vi "总磷总氮测量数据储存.vi"() -> ()   [LabVIEW 2022 SP3, in "斯坦道CODcr.lvlib"]
uses:
  <vilib>/ptbypt/NI_PtbyPt.lvlib
panel:
  in  "x":bool
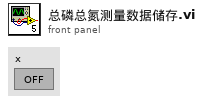
[diagram p1: front panel]
types:
  T1 = cluster{"跨度值":dbl, "零点标准液浓度":dbl, "跨度标准液浓度":dbl, "标准液标准浓度":dbl}
  T2 = cluster{"系统时间":timestamp, "工作状态":u16, "测量模式":enum16{"待机", "连续模式", "周期模式", "定点模式", "受控模式", "手动模式"}, "告警代码":u16, "故障代码":u16, "日志代码":u16, "软件版本":u16, "F0":sgl, "F1":sgl, "F2":sgl, "F3":sgl, "T":sgl, "H":sgl, "id":u16, "flowid":u16, "量程":u16, "总磷控温温度1":sgl, "营养盐控温温度2":sgl, "ADC":sgl, "结果值":sgl, "运行时间":u16, "步骤详情":string, "步骤流程":string}
  T3 = cluster{"运行模式":enum16{"维护模式", "常规模式", "应急模式", "质控模式", "性能测试"}, "质控频次":enum16{"关闭", "每天", "星期一", "星期二", "星期三", "星期四", "星期五", "星期六", "星期日"}, "空白核查时间":u16, "跨度核查时间":u16, "测量间隔":u16}
  T4 = cluster{"测量精度":u16, "消解温度":u16, "消解时长":u16, "量程下限":sgl, "量程上限":sgl, "曲线斜率K":sgl, "曲线斜率B":sgl, "标定日期":timestamp, "标液1浓度":sgl, "标液1测量过程值":sgl, "标液2浓度":sgl, "标液2测量过程值":sgl, "标液3浓度":sgl, "标液3测量过程值":sgl, "标液4浓度":sgl, "标液4测量过程值":sgl, "标液5浓度":sgl, "标液5测量过程值":sgl, "线性相关系数":sgl, "试剂余量":u32, "测量滴定值或吸光度":sgl, "空白校准时间":timestamp, "标样校准时间":timestamp, "检出限值":sgl, "校准系数":sgl, "设备系列号":string}[]
  T5 = cluster{"因子编码":u32, "单位":u16, "标样参考值":sgl, "水样数据时间":timestamp, "水样实测值":sgl, "水样数据标识":string, "标样数据时间":timestamp, "标样实测值":sgl, "标样数据标识":string, "空白数据时间":timestamp, "空白实测值":sgl, "空白数据标识":string, "零点核查数据时间":timestamp, "零点核查实测值":sgl, "零点核查数据标识":string, "跨度核查数据时间":timestamp, "跨度核查实测值":sgl, "跨度核查数据标识":string, "加标回收数据时间":timestamp, "加标回收实测值":sgl, "加标回收数据标识":string, "平行样数据时间":timestamp, "平行样实测值":sgl, "平行样数据标识":string, "F0":sgl, "F1":sgl, "F2":sgl, "F3":sgl, "F4":sgl, "F5":sgl, "F6":sgl, "F7":sgl, "温度":sgl, "湿度":sgl, "X值":sgl, "fidrange":u16, "X1值":sgl}[]
  T6 = cluster{"总磷跨度值":dbl, "总磷零点标准液浓度":dbl, "总磷跨度标准液浓度":dbl, "总磷标准液标准浓度":dbl, "总氮跨度值":dbl, "总氮零点标准液浓度":dbl, "总氮跨度标准液浓度":dbl, "总氮标准液标准浓度":dbl, "COD跨度值":dbl, "COD零点标准液浓度":dbl, "COD跨度标准液浓度":dbl, "COD标准液标准浓度":dbl, "氨氮跨度值":dbl, "氨氮零点标准液浓度":dbl, "氨氮跨度标准液浓度":dbl, "氨氮标准液标准浓度":dbl, "磷酸盐跨度值":dbl, "磷酸盐零点标准液浓度":dbl, "磷酸盐跨度标准液浓度":dbl, "磷酸盐标准液标准浓度":dbl, "硝氮跨度值":dbl, "硝氮零点标准液浓度":dbl, "硝氮跨度标准液浓度":dbl, "硝氮标准液标准浓度":dbl, "亚硝氮跨度值":dbl, "亚硝氮零点标准液浓度":dbl, "亚硝氮跨度标准液浓度":dbl, "亚硝氮标准液标准浓度":dbl, "硫化物跨度值":dbl, "硫化物零点标准液浓度":dbl, "硫化物跨度标准液浓度":dbl, "硫化物标准液标准浓度":dbl, "硅酸盐跨度值":dbl, "硅酸盐零点标准液浓度":dbl, "硅酸盐跨度标准液浓度":dbl, "硅酸盐标准液标准浓度":dbl, "总磷零点标准液偏差":dbl, "总磷跨度标准液偏差":dbl, "总磷标准液标准偏差":dbl, "总氮零点标准液偏差":dbl, "总氮跨度标准液偏差":dbl, "总氮标准液标准偏差":dbl, "COD零点标准液偏差":dbl, "COD跨度标准液偏差":dbl, "COD标准液标准偏差":dbl, "氨氮零点标准液偏差":dbl, "氨氮跨度标准液偏差":dbl, "氨氮标准液标准偏差":dbl, "磷酸盐零点标准液偏差":dbl, "磷酸盐跨度标准液偏差":dbl, "磷酸盐标准液标准偏差":dbl, "硝氮零点标准液偏差":dbl, "硝氮跨度标准液偏差":dbl, "硝氮标准液标准偏差":dbl, "亚硝氮零点标准液偏差":dbl, "亚硝氮跨度标准液偏差":dbl, "亚硝氮标准液标准偏差":dbl, "硫化物零点标准液偏差":dbl, "硫化物跨度标准液偏差":dbl, "硫化物标准液标准偏差":dbl, "硅酸盐零点标准液偏差":dbl, "硅酸盐跨度标准液偏差":dbl, "硅酸盐标准液标准偏差":dbl, "氟化物跨度值":dbl, "氟化物零点标准液浓度":dbl, "氟化物跨度标准液浓度":dbl, "氟化物标准液标准浓度":dbl, "氟化物零点标准液偏差":dbl, "氟化物跨度标准液偏差":dbl, "氟化物标准液标准偏差":dbl, "CODMn跨度值":dbl, "CODMn零点标准液浓度":dbl, "CODMn跨度标准液浓度":dbl, "CODMn标准液标准浓度":dbl, "CODMn零点标准液偏差":dbl, "CODMn跨度标准液偏差":dbl, "CODMn标准液标准偏差":dbl}
  T7 = enum16{"水样测试", "标样核查", "跨度核查", "零点核查", "加标回收", "空白测试", "平行样"}[]
  T8 = cluster{"因子编码":u32, "单位":u16, "标样参考值":sgl, "水样数据时间":timestamp, "水样实测值":sgl, "水样数据标识":string, "标样数据时间":timestamp, "标样实测值":sgl, "标样数据标识":string, "空白数据时间":timestamp, "空白实测值":sgl, "空白数据标识":string, "零点核查数据时间":timestamp, "零点核查实测值":sgl, "零点核查数据标识":string, "跨度核查数据时间":timestamp, "跨度核查实测值":sgl, "跨度核查数据标识":string, "加标回收数据时间":timestamp, "加标回收实测值":sgl, "加标回收数据标识":string, "平行样数据时间":timestamp, "平行样实测值":sgl, "平行样数据标识":string, "F0":sgl, "F1":sgl, "F2":sgl, "F3":sgl, "F4":sgl, "F5":sgl, "F6":sgl, "F7":sgl, "温度":sgl, "湿度":sgl, "X值":sgl, "fidrange":u16, "X1值":sgl}
  T9 = cluster{"时间标识":timestamp, "测量模式":enum16{"维护数据", "水样测试", "标样核查", "零点核查", "跨度核查", "空白测试", "平行样测试", "加标回收", "空白校准", "标样校准", "初始化（清洗）", "快捷测试"}, "数据标记表":string, "监测值":sgl, "单位":u16, "数据标识":string, "因子编码":u32, "标样参考值":sgl, "F0":sgl, "F1":sgl, "F2":sgl, "F3":sgl, "F4":sgl, "F5":sgl, "F6":sgl, "F7":sgl, "X":sgl, "温度":sgl, "湿度":sgl, "量程标识":string, "SN":string, "跨度值":sgl, "X1":sgl}
  T10 = typedef "斯坦道CODcr.lvlib/关键参数.ctl" = cluster{"测量量程":sgl, "测量检出限":sgl, "测量精度":sgl, "测量间隔":sgl, "消解温度":sgl, "消解时长":sgl, "三项式系数":sgl, "二次多项式系数":sgl, "曲线斜率":sgl, "曲线截距":sgl, "线性相关系数":sgl, "空白校准时间":timestamp, "标样校准时间":timestamp, "测量信号值":sgl, "稀释倍数":sgl, "空白标定系数":sgl, "量程系数":sgl}
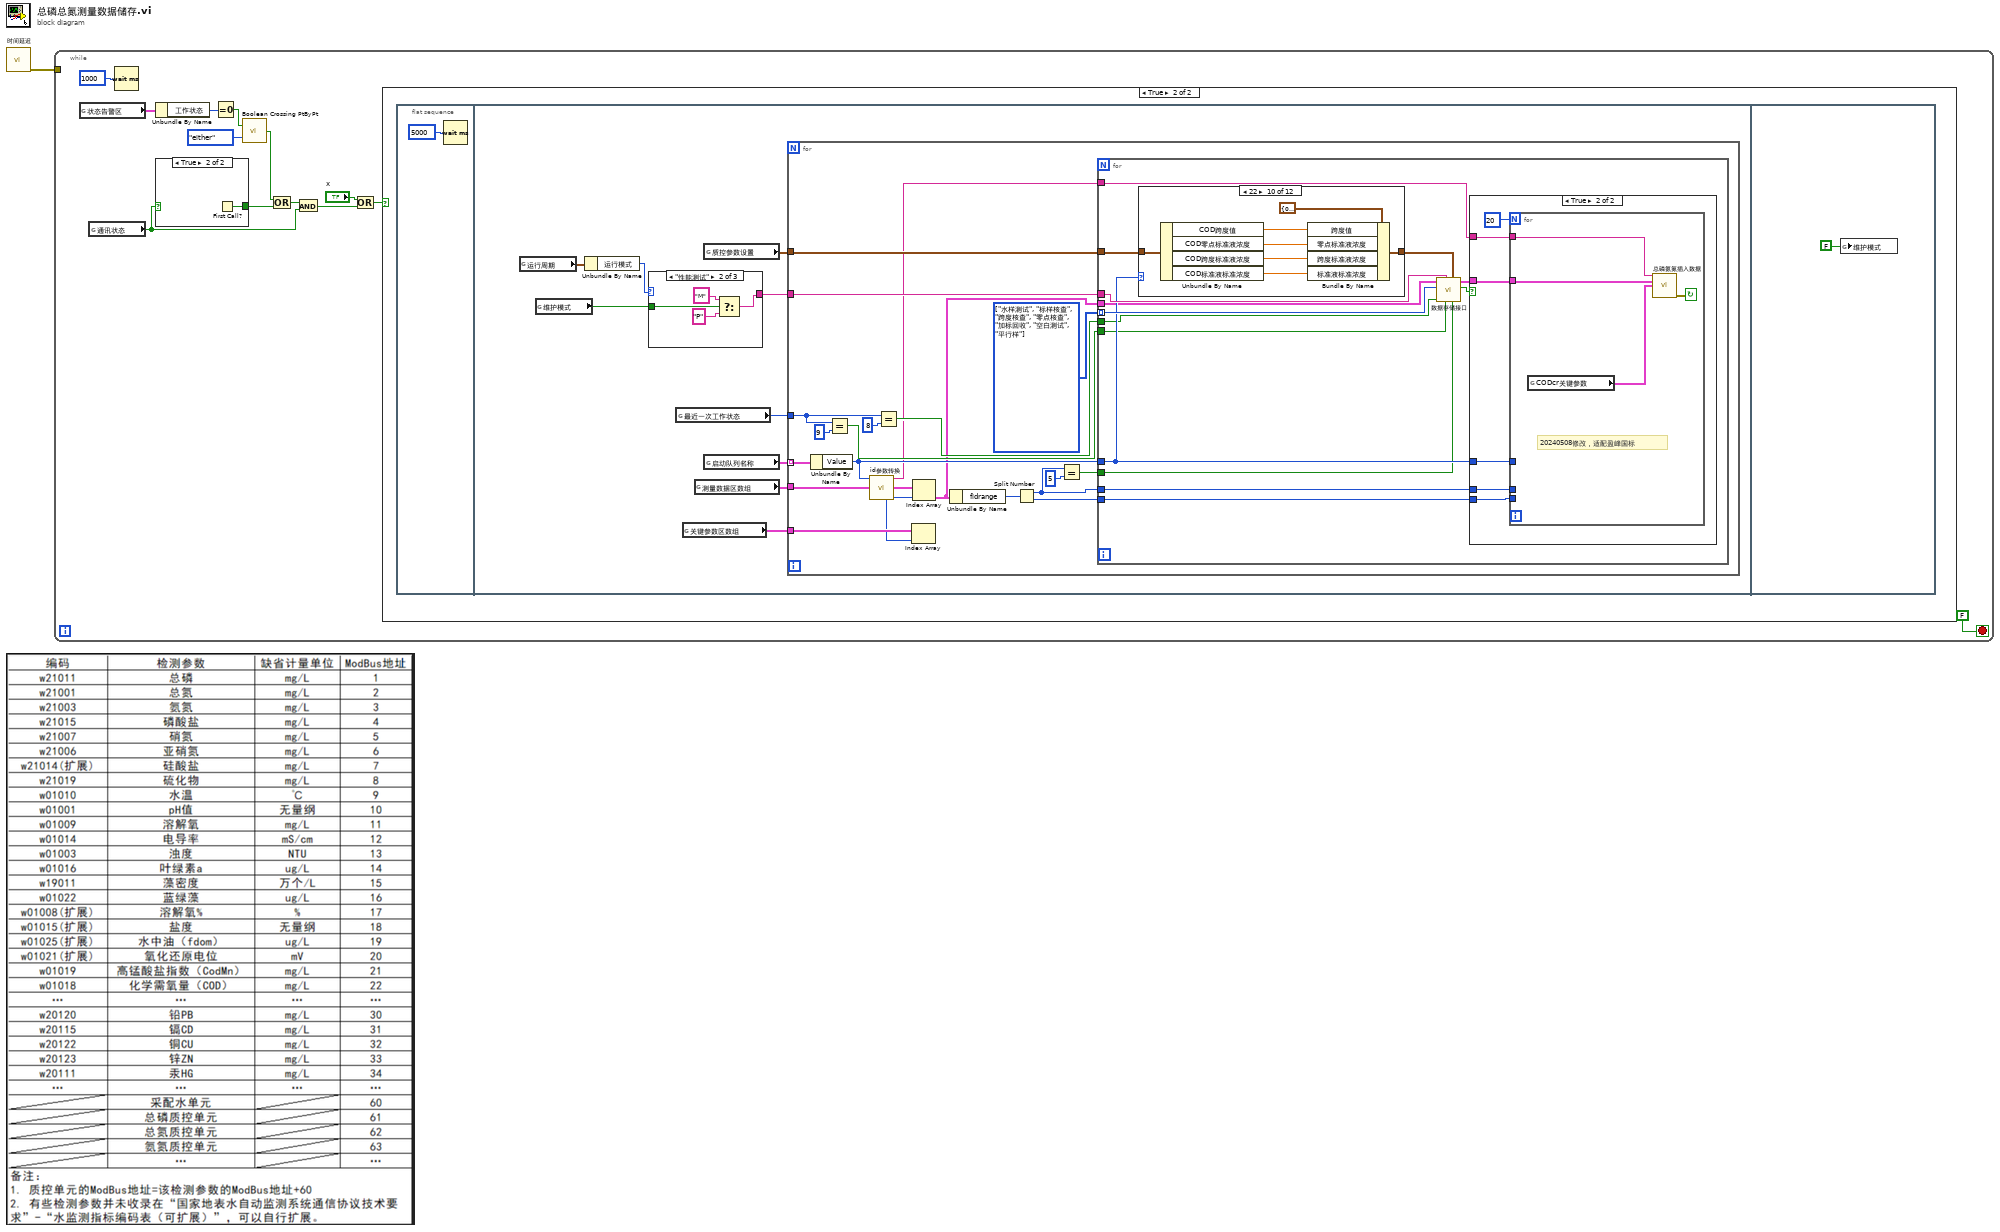
[diagram p0: block diagram]
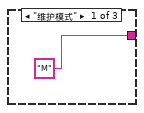
[diagram p4: hidden frame]
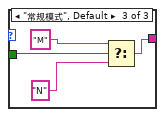
[diagram p5: hidden frame]
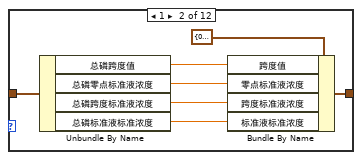
[diagram p8: hidden frame]
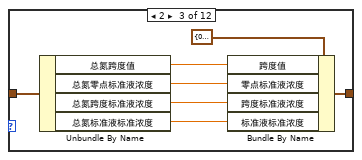
[diagram p9: hidden frame]
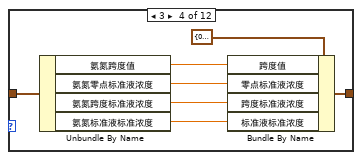
[diagram p10: hidden frame]
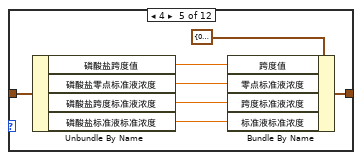
[diagram p11: hidden frame]
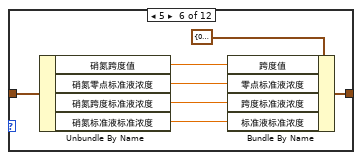
[diagram p12: hidden frame]
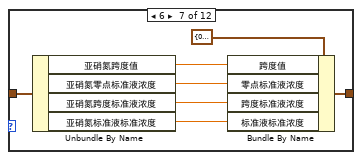
[diagram p13: hidden frame]
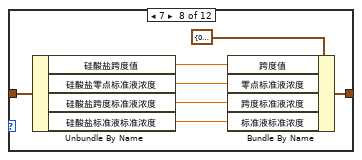
[diagram p14: hidden frame]
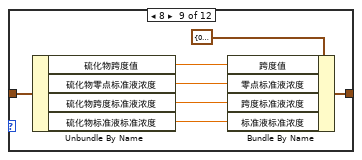
[diagram p15: hidden frame]
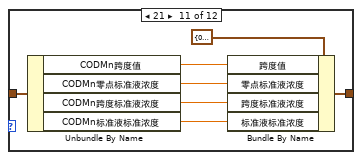
[diagram p16: hidden frame]
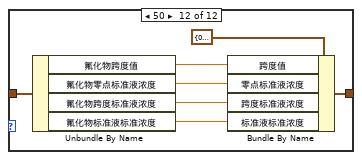
[diagram p17: hidden frame]
diagram:
  n1 = call "时间延迟"() -> ("error out"=w1:errorcluster)  [unwired: 11 in]
  n2 = while {
    tunnel: w1 -> [_]
    stop <- FALSE stop-if-true
    n3 = global read "VAR总磷总氮全局变量.vi" "状态告警区"() -> (w13:T2)
    n4 = global read "VAR总磷总氮全局变量.vi" "通讯状态"() -> (w6:bool)
    n5 = Wait (ms)(milliseconds to wait=u32 1000 ("等待时间（毫秒）")) -> ()  [unwired: 1 out]
    n6 = Unbundle By Name(w13) -> ("工作状态"=w11:u16)
    n7 = case shown="True" w6 {
      tunnel: [_ w15] -> w4
      frame False {
      }
      frame True {
        n8 = First Call?() -> (First Call?: T/F=w15:bool)
      }
    }
    n9 = Equal To 0?(x=w11) -> (x = 0?=w8:bool)
    n10 = call <vilib>:"Boolean Crossing PtByPt.vi"("direction"=enum16{"either", "false-true", "true-false"}."either", "input"=w8) -> ("crossing"=w9:bool)  [unwired: 1 in]
    n11 = Or(x=w9, y=w4) -> (x .or. y?=w5:bool)
    n12 = And(x=w5, y=w6) -> (x .and. y?=w7:bool)
    n13 = Or(x="x", y=w7) -> (x .or. y?=w3:bool)
    n14 = case shown="True" w3 {
      frame False {
      }
      frame True {
        n15 = flat-sequence {
          frame #0 {
            n16 = Wait (ms)(milliseconds to wait=u32 5000 ("等待时间（毫秒）")) -> ()  [unwired: 1 out]
          }
          frame #1 {
            n17 = global read "总磷总氮断电保存全局变量.vi" "运行周期"() -> (w22:T3)
            n18 = global read "VAR总磷总氮全局变量.vi" "维护模式"() -> (w19:bool)
            n19 = Unbundle By Name(w22) -> ("运行模式"=w20:enum16{"维护模式", "常规模式", "应急模式", "质控模式", "性能测试"})
            n20 = case shown="\"性能测试\"" w20 {
              tunnel: ["M" w27 w32] -> w21
              tunnel: w19 -> [_ w28 w34]
              frame "维护模式" {
              }
              frame "性能测试" {
                n21 = Select(t="M", s=w28, f="P") -> (s? t:f=w27:string)
              }
              frame "常规模式", Default {
                n22 = Select(t="M", s=w34, f="N") -> (s? t:f=w32:string)
              }
            }
            n23 = global read "VAR总磷总氮全局变量.vi" "最近一次工作状态"() -> (w24:u16)
            n24 = global read "VAR总磷总氮全局变量.vi" "关键参数区数组"() -> (w17:T4)
            n25 = global read "VAR总磷总氮全局变量.vi" "测量数据区数组"() -> (w18:T5)
            n26 = global read "总磷总氮断电保存全局变量.vi" "质控参数设置"() -> (w23:T6)
            n27 = global read "model config var.vi" "启动队列名称"() -> (w25:cluster{"String":string, "Value":u16}[])
            n28 = for {
              tunnel: w25 -> [w51] mode=indexing
              tunnel: w24 -> [w47]
              tunnel: w23 -> [w53]
              tunnel: w21 -> [w52]
              tunnel: w18 -> [w37]
              tunnel: w17 -> [w36]
              w54 = T7 [enum."水样测试", enum."标样核查", enum."跨度核查", enum."零点核查", enum."加标回收", enum."空白测试", enum."平行样"] items=["水样测试", "标样核查", "跨度核查", "零点核查", "加标回收", "空白测试", "平行样"]
              n29 = Unbundle By Name(w51) -> ("Value"=w45:u16)
              n30 = Equal?(x=w47, y=u16 9) -> (x = y?=w46:bool)
              n31 = call "id参数转换.vi"("id"=w45) -> ("table输出"=w44:string, "数组资源索引"=w35:i32)  [unwired: 9 in]
              n32 = Equal?(x=w47, y=u16 8) -> (x = y?=w49:bool)
              n33 = Index Array(array=w36, index=w35) -> ()  [unwired: 1 out]
              n34 = Index Array(array=w37, index=w35) -> (element=w41:T8)
              n35 = Unbundle By Name(w41) -> ("fidrange"=w43:u16)
              n36 = Split Number(x=w43) -> (hi(x)=w38:u8, lo(x)=w39:u8)
              n37 = Equal?(x=w38, y=u16 5) -> (x = y?=w40:bool)
              n38 = for {
                tunnel: w54 -> [w66] mode=indexing
                tunnel: w53 -> [w65]
                tunnel: w52 -> [w64]
                tunnel: w45 -> [w63]
                tunnel: w49 -> [w62]
                tunnel: w46 -> [w61]
                tunnel: w41 -> [w56]
                tunnel: w44 -> [w60]
                tunnel: w40 -> [w59]
                tunnel: w39 -> [w58]
                tunnel: w38 -> [w57]
                n39 = case shown="22" w63 {
                  tunnel: w65 -> [_ w85 w92 w99 w106 w113 w120 w127 w134 w141 w148 w155]
                  tunnel: [_ w83 w90 w97 w104 w111 w118 w125 w132 w139 w146 w153] -> w67
                  frame 0, Default {
                  }
                  frame 1 {
                    n40 = Unbundle By Name(w85) -> ("总磷跨度值"=w82:dbl, "总磷零点标准液浓度"=w81:dbl, "总磷跨度标准液浓度"=w80:dbl, "总磷标准液标准浓度"=w79:dbl)
                    n41 = Bundle By Name(cluster=T1 {"跨度值"=0.0, "零点标准液浓度"=0.0, "跨度标准液浓度"=0.0, "标准液标准浓度"=0.0} ("质控参数设置"), "跨度值"=w82, "零点标准液浓度"=w81, "跨度标准液浓度"=w80, "标准液标准浓度"=w79) -> (w83:T1)
                  }
                  frame 2 {
                    n42 = Unbundle By Name(w92) -> ("总氮跨度值"=w89:dbl, "总氮零点标准液浓度"=w88:dbl, "总氮跨度标准液浓度"=w87:dbl, "总氮标准液标准浓度"=w86:dbl)
                    n43 = Bundle By Name(cluster=T1 {"跨度值"=0.0, "零点标准液浓度"=0.0, "跨度标准液浓度"=0.0, "标准液标准浓度"=0.0} ("质控参数设置"), "跨度值"=w89, "零点标准液浓度"=w88, "跨度标准液浓度"=w87, "标准液标准浓度"=w86) -> (w90:T1)
                  }
                  frame 3 {
                    n44 = Unbundle By Name(w99) -> ("氨氮跨度值"=w96:dbl, "氨氮零点标准液浓度"=w95:dbl, "氨氮跨度标准液浓度"=w94:dbl, "氨氮标准液标准浓度"=w93:dbl)
                    n45 = Bundle By Name(cluster=T1 {"跨度值"=0.0, "零点标准液浓度"=0.0, "跨度标准液浓度"=0.0, "标准液标准浓度"=0.0} ("质控参数设置"), "跨度值"=w96, "零点标准液浓度"=w95, "跨度标准液浓度"=w94, "标准液标准浓度"=w93) -> (w97:T1)
                  }
                  frame 4 {
                    n46 = Unbundle By Name(w106) -> ("磷酸盐跨度值"=w103:dbl, "磷酸盐零点标准液浓度"=w102:dbl, "磷酸盐跨度标准液浓度"=w101:dbl, "磷酸盐标准液标准浓度"=w100:dbl)
                    n47 = Bundle By Name(cluster=T1 {"跨度值"=0.0, "零点标准液浓度"=0.0, "跨度标准液浓度"=0.0, "标准液标准浓度"=0.0} ("质控参数设置"), "跨度值"=w103, "零点标准液浓度"=w102, "跨度标准液浓度"=w101, "标准液标准浓度"=w100) -> (w104:T1)
                  }
                  frame 5 {
                    n48 = Unbundle By Name(w113) -> ("硝氮跨度值"=w110:dbl, "硝氮零点标准液浓度"=w109:dbl, "硝氮跨度标准液浓度"=w108:dbl, "硝氮标准液标准浓度"=w107:dbl)
                    n49 = Bundle By Name(cluster=T1 {"跨度值"=0.0, "零点标准液浓度"=0.0, "跨度标准液浓度"=0.0, "标准液标准浓度"=0.0} ("质控参数设置"), "跨度值"=w110, "零点标准液浓度"=w109, "跨度标准液浓度"=w108, "标准液标准浓度"=w107) -> (w111:T1)
                  }
                  frame 6 {
                    n50 = Unbundle By Name(w120) -> ("亚硝氮跨度值"=w117:dbl, "亚硝氮零点标准液浓度"=w116:dbl, "亚硝氮跨度标准液浓度"=w115:dbl, "亚硝氮标准液标准浓度"=w114:dbl)
                    n51 = Bundle By Name(cluster=T1 {"跨度值"=0.0, "零点标准液浓度"=0.0, "跨度标准液浓度"=0.0, "标准液标准浓度"=0.0} ("质控参数设置"), "跨度值"=w117, "零点标准液浓度"=w116, "跨度标准液浓度"=w115, "标准液标准浓度"=w114) -> (w118:T1)
                  }
                  frame 7 {
                    n52 = Unbundle By Name(w127) -> ("硅酸盐跨度值"=w124:dbl, "硅酸盐零点标准液浓度"=w123:dbl, "硅酸盐跨度标准液浓度"=w122:dbl, "硅酸盐标准液标准浓度"=w121:dbl)
                    n53 = Bundle By Name(cluster=T1 {"跨度值"=0.0, "零点标准液浓度"=0.0, "跨度标准液浓度"=0.0, "标准液标准浓度"=0.0} ("质控参数设置"), "跨度值"=w124, "零点标准液浓度"=w123, "跨度标准液浓度"=w122, "标准液标准浓度"=w121) -> (w125:T1)
                  }
                  frame 8 {
                    n54 = Unbundle By Name(w134) -> ("硫化物跨度值"=w131:dbl, "硫化物零点标准液浓度"=w130:dbl, "硫化物跨度标准液浓度"=w129:dbl, "硫化物标准液标准浓度"=w128:dbl)
                    n55 = Bundle By Name(cluster=T1 {"跨度值"=0.0, "零点标准液浓度"=0.0, "跨度标准液浓度"=0.0, "标准液标准浓度"=0.0} ("质控参数设置"), "跨度值"=w131, "零点标准液浓度"=w130, "跨度标准液浓度"=w129, "标准液标准浓度"=w128) -> (w132:T1)
                  }
                  frame 22 {
                    n56 = Unbundle By Name(w141) -> ("COD跨度值"=w138:dbl, "COD零点标准液浓度"=w137:dbl, "COD跨度标准液浓度"=w136:dbl, "COD标准液标准浓度"=w135:dbl)
                    n57 = Bundle By Name(cluster=T1 {"跨度值"=0.0, "零点标准液浓度"=0.0, "跨度标准液浓度"=0.0, "标准液标准浓度"=0.0} ("质控参数设置"), "跨度值"=w138, "零点标准液浓度"=w137, "跨度标准液浓度"=w136, "标准液标准浓度"=w135) -> (w139:T1)
                  }
                  frame 21 {
                    n58 = Unbundle By Name(w148) -> ("CODMn跨度值"=w145:dbl, "CODMn零点标准液浓度"=w144:dbl, "CODMn跨度标准液浓度"=w143:dbl, "CODMn标准液标准浓度"=w142:dbl)
                    n59 = Bundle By Name(cluster=T1 {"跨度值"=0.0, "零点标准液浓度"=0.0, "跨度标准液浓度"=0.0, "标准液标准浓度"=0.0} ("质控参数设置"), "跨度值"=w145, "零点标准液浓度"=w144, "跨度标准液浓度"=w143, "标准液标准浓度"=w142) -> (w146:T1)
                  }
                  frame 50 {
                    n60 = Unbundle By Name(w155) -> ("氟化物跨度值"=w152:dbl, "氟化物零点标准液浓度"=w151:dbl, "氟化物跨度标准液浓度"=w150:dbl, "氟化物标准液标准浓度"=w149:dbl)
                    n61 = Bundle By Name(cluster=T1 {"跨度值"=0.0, "零点标准液浓度"=0.0, "跨度标准液浓度"=0.0, "标准液标准浓度"=0.0} ("质控参数设置"), "跨度值"=w152, "零点标准液浓度"=w151, "跨度标准液浓度"=w150, "标准液标准浓度"=w149) -> (w153:T1)
                  }
                }
                n62 = call "数据存储接口.vi"("快捷测试？"=w59, "质控参数设置"=w67, "标样校准？"=w61, "数据标记表"=w64, "空白校准？"=w62, "数据存储模式"=w66, "测量数据区"=w56) -> ("x != y?"=w55:bool, "data输出"=w68:T9)  [unwired: 3 in]
                n63 = case shown="True" w55 {
                  tunnel: w68 -> [_ w74]
                  tunnel: w63 -> [_ w73]
                  tunnel: w60 -> [_ w72]
                  tunnel: w58 -> [_ w71]
                  tunnel: w57 -> [_ w70]
                  frame False {
                  }
                  frame True {
                    n64 = for {
                      N: 20 -> [_]
                      tunnel: w74 -> [w78]
                      tunnel: w73 -> [_]
                      tunnel: w72 -> [w77]
                      tunnel: w71 -> [_]
                      tunnel: w70 -> [_]
                      stop <- w76 continue-if-true
                      # "20240508修改，适配盈峰国标"
                      n65 = global read "VAR总磷总氮全局变量.vi" "CODcr关键参数"() -> (w75:T10)
                      n66 = call "总磷氨氮插入数据.vi"("table"=w77, "data"=w78, "关键参数"=w75) -> ("error out"=w76:errorcluster)  [unwired: 12 in]
                    }
                  }
                }
              }
            }
          }
          frame #2 {
            n67 = global write "VAR总磷总氮全局变量.vi" "维护模式"(FALSE ("维护模式")) -> ()
          }
        }
      }
    }
  }
